vi "ChipScope Control.vi"() -> ()   [LabVIEW 2017]
uses:
  <instrlib>/TLDC4100/TLDC4100.llb/z_StateMachineVorlage.ctl
  C:/Program Files/National Instruments/LabVIEW 2017/instr.lib/IDS/ueye.NET/uEyeDotNet.dll
panel:
  in  "Acquisition tab":enum32{"Acquisition", "Bookmarks"}(tab)
  in  "Exposure 3":dbl=100.0
  in  "Exposure 2":dbl=100.0
  in  "Gain 3":i32=100 min=100 max=2000
  in  "Gain 2":i32=100 min=100 max=2000
  in  "Gain 1":i32=100 caption="Gain" min=100 max=2000
  in  "Exposure 1":dbl=100.0 caption="Exp."
  in  "Acq. order":string(combo)="3"
  in  "ACQUIRE":bool
  in  "Autosave?":bool
  in  "Use bookmarks?":bool
  in  "t-delay (ms)":dbl min=0.0 max=75.0
  in  "# t-frames":i32=1 min=0 max=75
  in  "z-step (um)":dbl=1.0 min=0.0 max=75.0
  in  "# z-steps":i32=1 min=0 max=75
  in  "3:":string(combo)="99"
  in  "2:":string(combo)="99"
  in  "1:":string(combo)="0"
  in  "Illumination tab":enum32{"Laser power", "LED power"}(tab)
  in  "Red power":dbl=1.0 min=0.0 max=120.0
  in  "Green power":dbl=1.0 min=0.0 max=150.0
  in  "Blue power":dbl=1.0 min=0.0 max=150.0
  in  "445 power":dbl=1.0 min=0.0 max=75.0
  in  "Illumination":bool
  out "Live":bool
  in  "Gain":i32=100 min=100 max=2000
  in  "Exposure (ms)":dbl=100.0
  in  "Live channel":enum8{"Red", "Green", "Blue"}(ring)
  in  "LIVE":bool
  out "Image":T1(plugin-control)
  out "Status":string
  out "Connected":bool
  out "error out":errorcluster
  in  "Quit":bool
  in  "error in":errorcluster
  out "State":T2 caption="States"
  # "Laser"
  # "LEDs"
  # "Laser power"
  # "Debugging area"
  # "Channel order"
  # "Acquisition order"
  # "LEDs seem to have a\nproblem with the \ndriver hardware at the\nmoment!! :("
  # "mW"
  # "mW"
  # "mW"
  # "mW"
  # "LEDs seem to have a\nproblem with the \ndriver hardware at the\nmoment!! :("
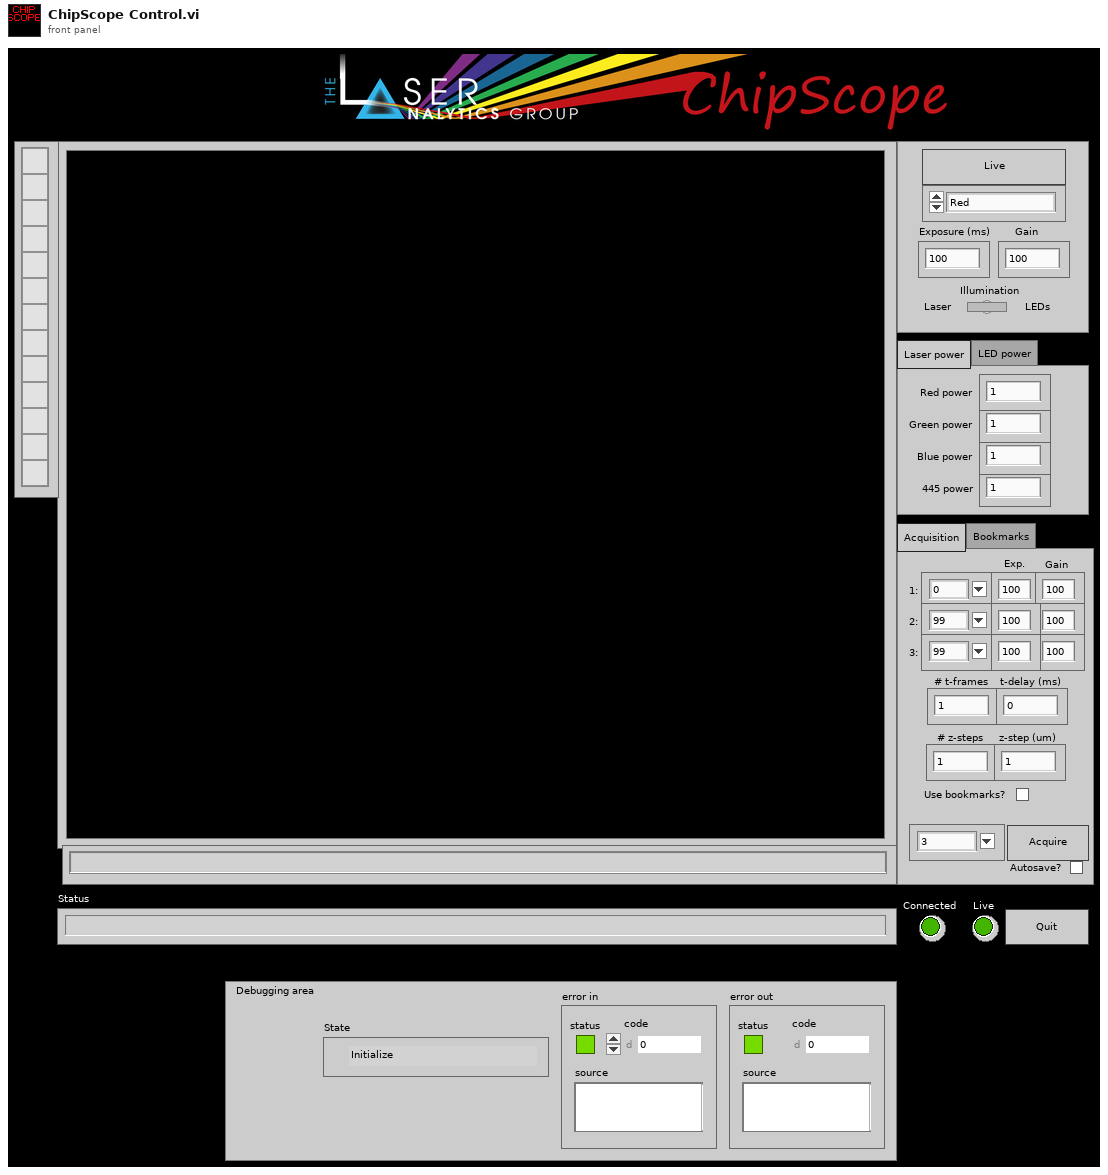
[diagram p1: front panel]
types:
  T1 = typedef "IMAQ Image.ctl" = refnum<image>
  T2 = typedef "z_StateMachineVorlage.ctl" = enum16{"Initialize", "1", "2", "3", "4", "5", "6", "7", "8", "9", "10", "11", "12", "13", "14", "15", "20", "25", "30", "35", "40", "45", "50", "55", "59", "60", "65", "70", "75", "76", "77", "78", "79", "80", "85", "90", "91", "92", "93", "94", "95", "96", "97", "98", "99", "100", "105", "110", "120", "130", "140", "150", "160", "170", "180", "190", "200", "201", "205", "210", "215", "220", "230", "240", "245", "250", "255", "260", "270", "280", "290", "300", "310", "313", "315", "318", "320", "330", "340", "350", "360", "370", "380", "390", "400", "410", "420", "430", "440", "450", "460", "470", "480", "490", "500", "501", "502", "510", "520", "523", "525", "528", "530", "540", "550", "560", "570", "580", "590", "600", "605", "610", "620", "630", "640", "650", "660", "670", "680", "690", "700", "710", "720", "730", "740", "750", "760", "770", "780", "790", "800", "810", "820", "830", "840", "850", "860", "870", "880", "890", "900", "910", "920", "930", "940", "950", "960", "970", "980", "990", "1000", "1010", "1020", "1030", "1040", "1050", "1060", "1070", "1080", "1090", "1100", "1110", "1120", "1130", "1140", "1150", "1160", "1170", "1180", "1190", "1200", "1210", "1220", "1230", "1240", "1250", "1260", "1270", "1280", "1290", "1300", "1310", "1320", "1330", "1340", "1350", "1360", "1370", "1380", "1390", "1400", "1410", "1420", "1430", "1440", "1450", "1460", "1470", "1480", "1490", "1500", "Fehler I", "Fehler II", "Fehler III", "Fehler IV", "Fehler V", "Fehler VI", "Fehler VII", "Fehler VIII", "Fehler IX", "Fehler X", "Stop"}
  T3 = cluster{"Save path":path, "t frame":i32, "bookmark #":i32, "Z-step":i32, "Channel":i32, "total t frames":i32, "Total bookmarks":i32, "Total z steps":i32, "Total channels":i32}
  T4 = cluster{"LED handle":refnum<visa-resource-name>, "Laser cluster":cluster{"445 laser":refnum<visa-resource-name>, "488 laser":refnum<visa-resource-name>, "561 laser":refnum<visa-resource-name>, "640 laser":refnum<visa-resource-name>}, "Piezo handle":i32, "Camera cluster":cluster{"Red camera":refnum<k24>, "Green camera":refnum<k24>, "Blue camera":refnum<k24>}}
  T5 = cluster{"445 laser":refnum<visa-resource-name>, "488 laser":refnum<visa-resource-name>, "561 laser":refnum<visa-resource-name>, "640 laser":refnum<visa-resource-name>}
  T6 = cluster{"Red camera":refnum<k24>, "Green camera":refnum<k24>, "Blue camera":refnum<k24>}
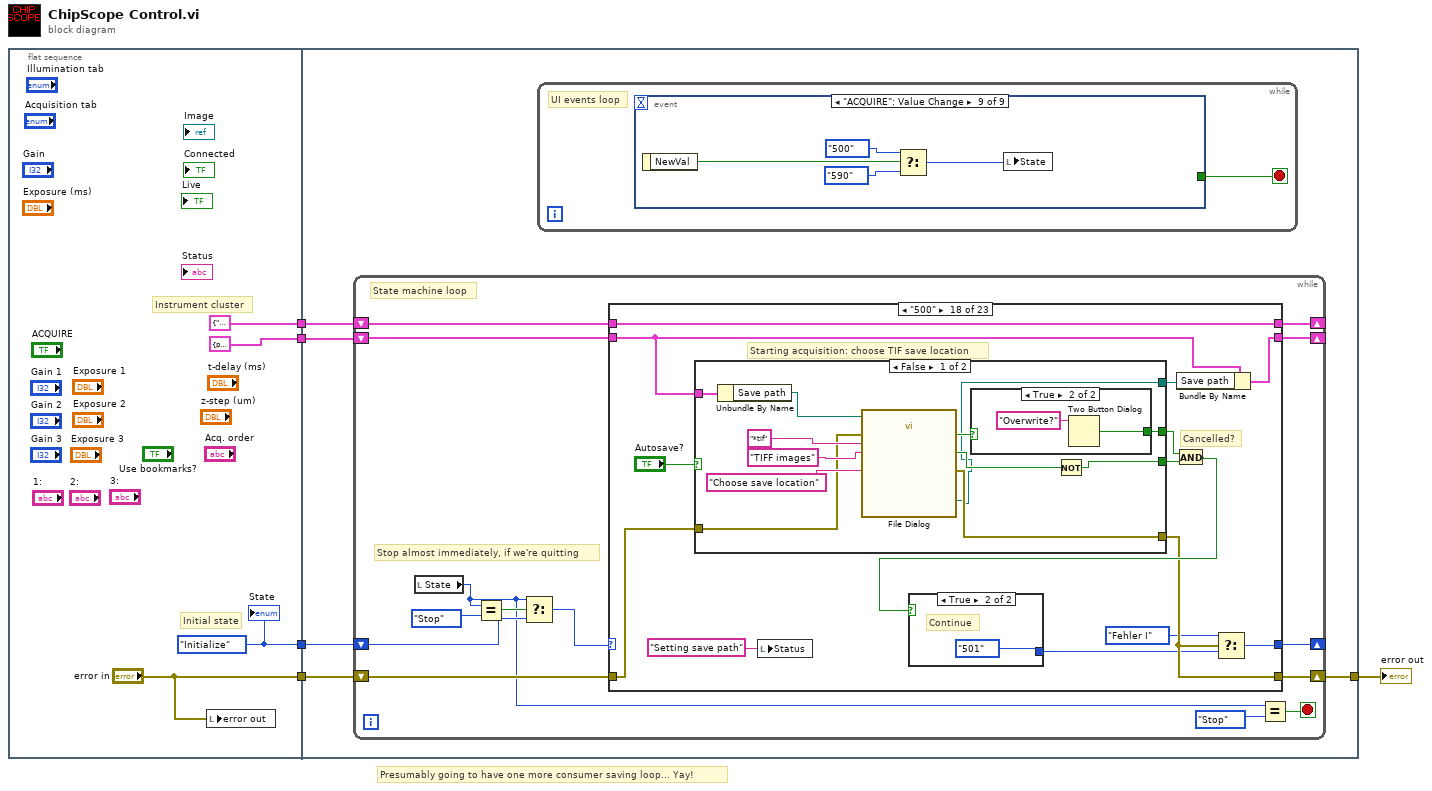
[diagram p0: block diagram]
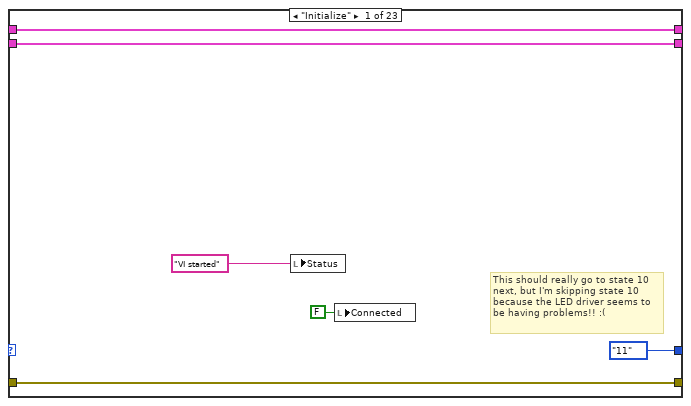
[diagram p2: hidden frame]
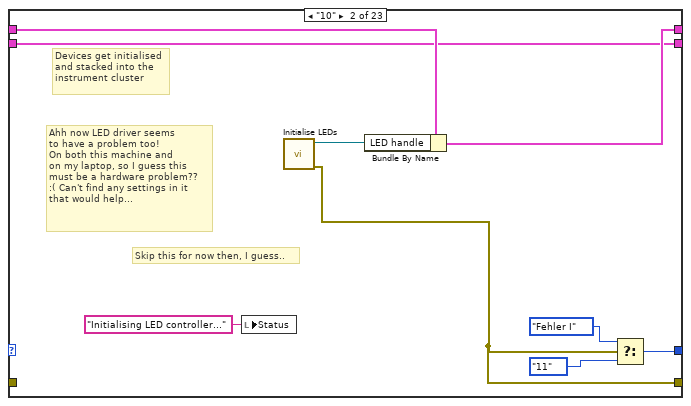
[diagram p3: hidden frame]
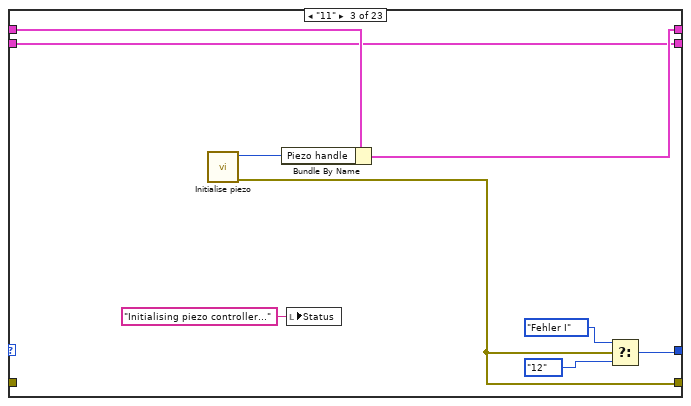
[diagram p4: hidden frame]
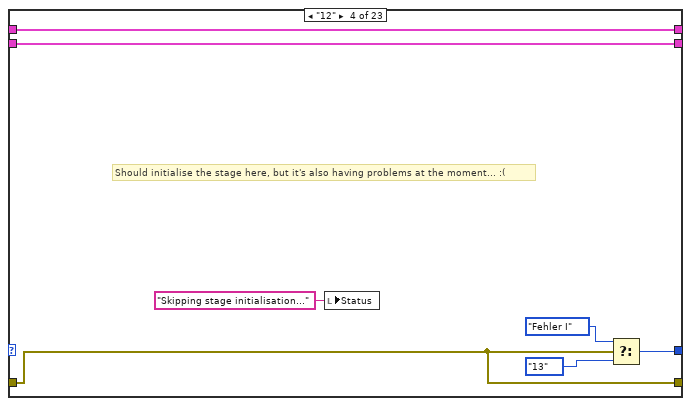
[diagram p5: hidden frame]
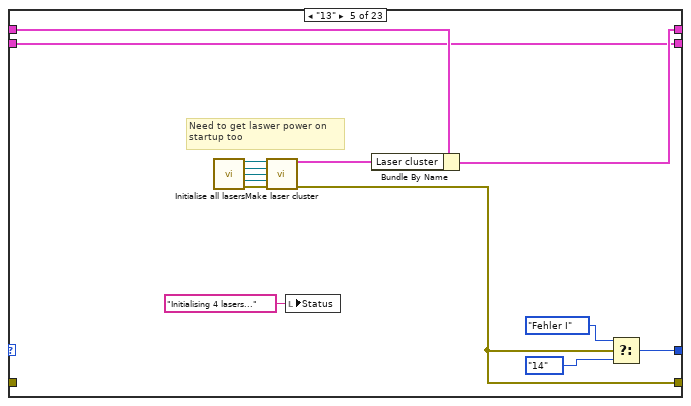
[diagram p6: hidden frame]
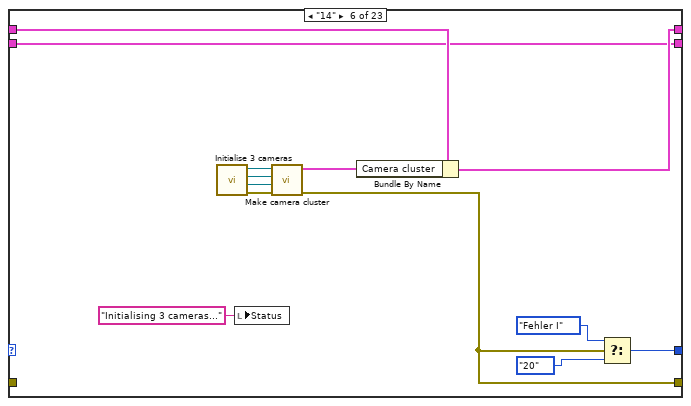
[diagram p7: hidden frame]
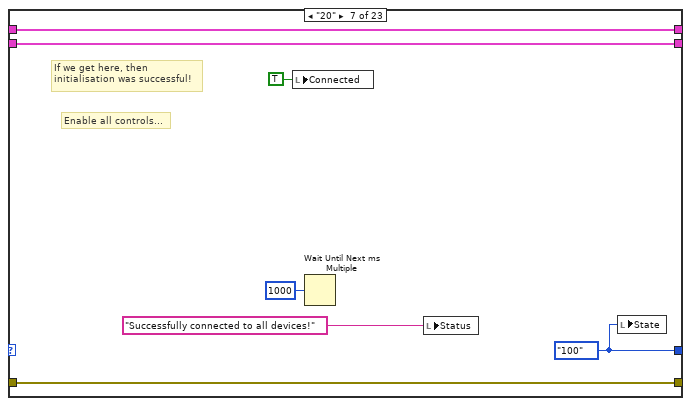
[diagram p8: hidden frame]
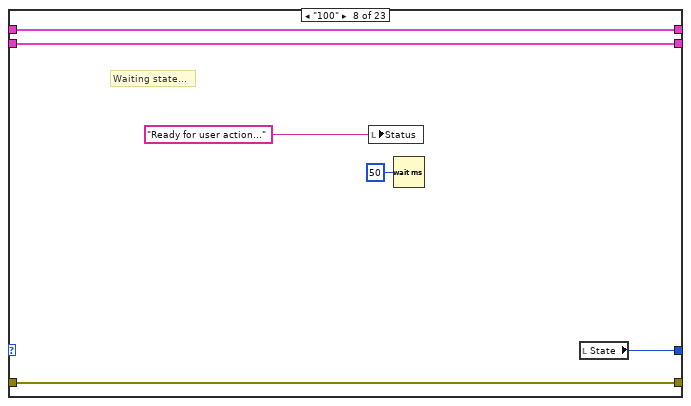
[diagram p9: hidden frame]
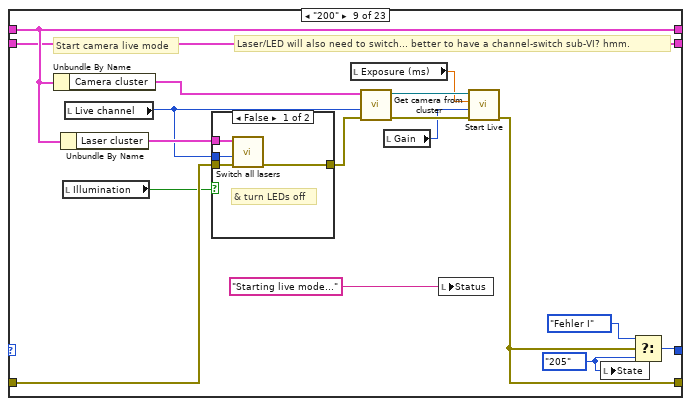
[diagram p10: hidden frame]
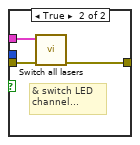
[diagram p11: hidden frame]
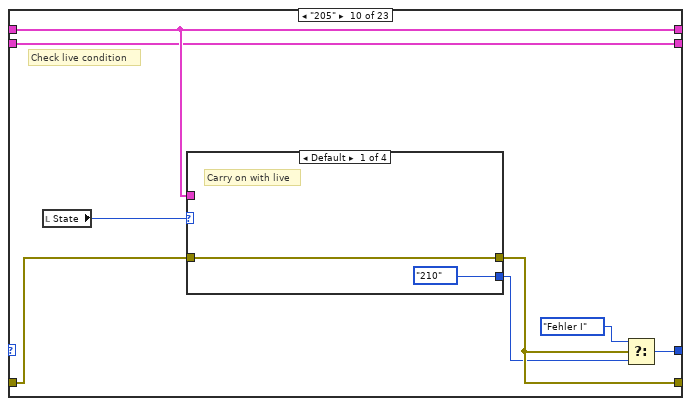
[diagram p12: hidden frame]
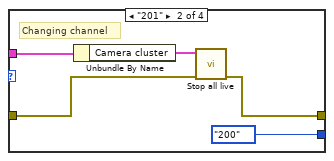
[diagram p13: hidden frame]
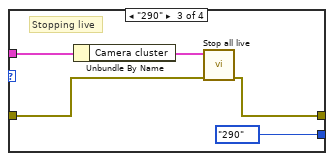
[diagram p14: hidden frame]
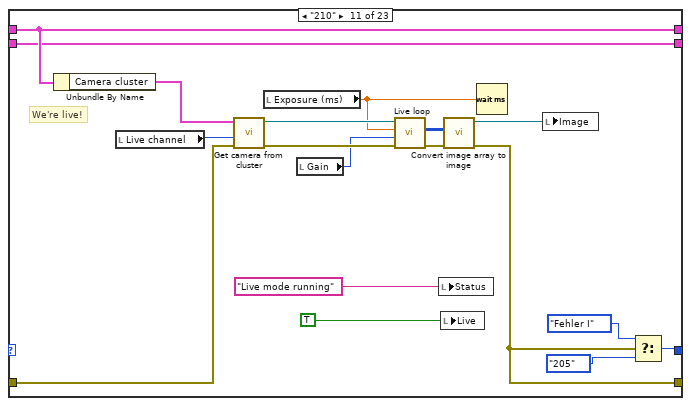
[diagram p16: hidden frame]
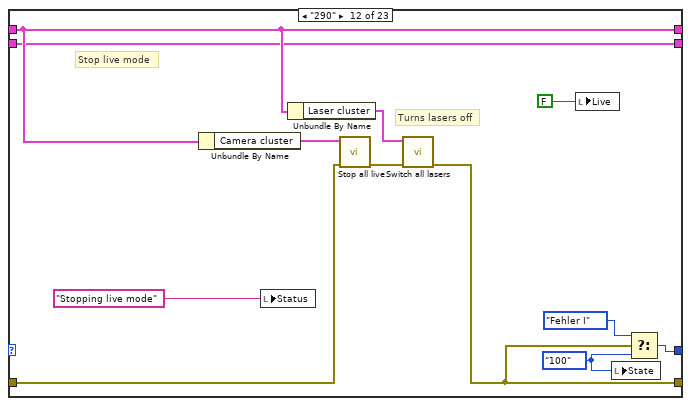
[diagram p17: hidden frame]
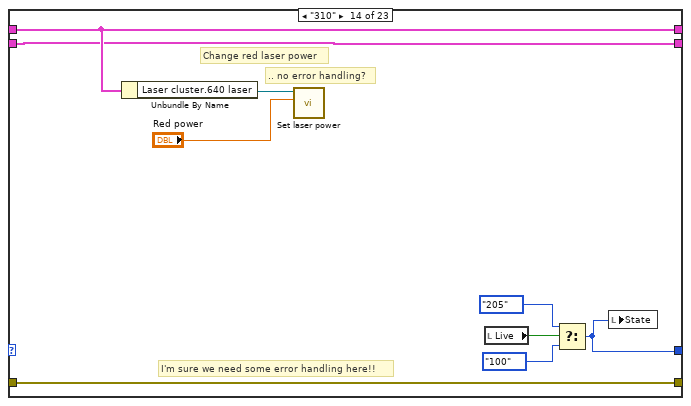
[diagram p19: hidden frame]
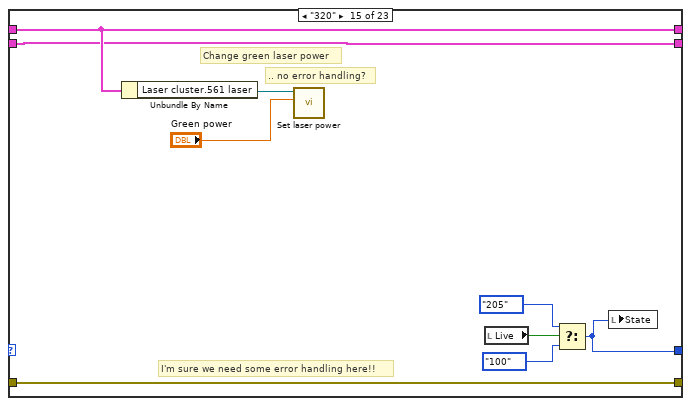
[diagram p20: hidden frame]
diagram:
  # "Presumably going to have one more consumer saving loop... Yay!"
  n1 = flat-sequence {
    tunnel: [T4 {"LED handle"="", "Laser cluster"={"445 laser"="", "488 laser"="", "561 laser"="", "640 laser"=""}, "Piezo handle"=0, "Camera cluster"={"Red camera"=refnum, "Green camera"=refnum, "Blue camera"=refnum}} ("Instrument cluster")] -> w5
    tunnel: ["error in"] -> w3
    tunnel: [w7] -> w2
    tunnel: [T3 {"Save path"=path "D:/DATA_2018", "t frame"=0, "bookmark #"=0, "Z-step"=0, "Channel"=0, "total t frames"=0, "Total bookmarks"=0, "Total z steps"=0, "Total channels"=0} ("Instrument cluster")] -> w1
    tunnel: w5 -> [w14]
    tunnel: [w13] -> w4
    tunnel: w3 -> [w12]
    tunnel: w2 -> [w11]
    tunnel: w1 -> [w10]
    frame #0 {
      w7 = z_StateMachineVorlage."Initialize" ("States")
      # "Initial state"
      # "Instrument cluster"
      n2 = local write "error out"("error in") -> ()
      "State" <- w7
    }
    frame #1 {
      n3 = while {
        shift-right: [w28] -> _
        shift-left: w11 -> [w18]
        shift-right: [w25] -> _
        shift-left: w14 -> [w22]
        shift-right: [w24] -> w13
        shift-left: w12 -> [w23]
        shift-right: [w16] -> _
        shift-left: w10 -> [w15]
        stop <- w27 stop-if-true
        # "State machine loop"
        # "Stop almost immediately, if we're quitting"
        n4 = local read "State"() -> (w17:T2)
        n5 = Equal?(x=w17, y=z_StateMachineVorlage."Stop" ("States")) -> (x = y?=w20:bool)
        n6 = Select(t=w17, s=w20, f=w18) -> (s? t:f=w19:T2)
        n7 = case shown="\"500\"" w19 {
          selector: w19 -> [_ _ _ _ _ _ _ _ _ _ _ _ w179 _ _ _ _ _ _ _ w290 _ _]
          tunnel: [z_StateMachineVorlage."11" ("States") w41 w47 w56 w62 w75 w88 w95 w114 w128 w160 w172 w179 w181 w191 w200 w209 w221 z_StateMachineVorlage."502" ("States") _ w290 z_StateMachineVorlage."Stop" ("States") z_StateMachineVorlage."900" ("States")] -> w28
          tunnel: [w31 w37 w51 w54 w64 w79 w90 w99 w106 w131 w163 w166 w177 w188 w197 w206 w215 w229 w261 w284 w289 w296 w302] -> w25
          tunnel: w22 -> [w31 w36 w50 w54 w65 w80 w90 w99 w106 w131 w163 w166 w177 w188 w197 w206 w215 w229 w261 w284 w289 w296 w302]
          tunnel: [w32 w39 w46 w55 w63 w76 w91 w97 w115 w127 w149 w168 w178 w182 w192 w201 w210 w223 w250 w276 w291 w293 w311] -> w24
          tunnel: w23 -> [w32 _ _ w55 _ _ w91 w97 w103 w130 w157 w175 w178 w182 w192 w201 w210 w227 w250 w276 w291 w294 w300]
          tunnel: w15 -> [w29 w35 w44 w53 w60 w74 w87 w94 w100 w124 w146 w164 w176 w180 w189 w198 w207 w218 w265 w285 w288 w292 w297]
          tunnel: [w29 w35 w44 w53 w60 w74 w87 w94 w100 w124 w146 w164 w176 w180 w189 w198 w207 w217 w253 w277 w288 w292 w297] -> w16
          frame "Initialize" {
            # "This should really go to state 10\nnext, but I'm skipping state 10\nbecause the LED driver seems to\nbe having problems!! :("
            n8 = local write "Status"("VI started" ("Status")) -> ()
            n9 = local write "Connected"(FALSE ("Connected")) -> ()
          }
          frame "10" {
            # "Skip this for now then, I guess.."
            # "Ahh now LED driver seems\nto have a problem too!\nOn both this machine and \non my laptop, so I guess this\nmust be a hardware problem??\n:( Can't find any settings in it \nthat would help..."
            # "Devices get initialised\nand stacked into the\ninstrument cluster"
            n10 = local write "Status"("Initialising LED controller..." ("Status")) -> ()
            n11 = call "Initialise LEDs.vi"() -> ("error out"=w39:errorcluster, "LED handle"=w38:refnum<visa-resource-name>)  [unwired: 10 in]
            n12 = Bundle By Name(cluster=w36, "LED handle"=w38) -> (w37:T4)
            n13 = Select(t=z_StateMachineVorlage."Fehler I", s=w39, f=z_StateMachineVorlage."11" ("States")) -> (s? t:f=w41:T2)
          }
          frame "11" {
            n14 = call "Initialise piezo.vi"() -> ("Piezo error out"=w46:errorcluster, "Piezo handle"=w52:i32)  [unwired: 10 in]
            n15 = Bundle By Name(cluster=w50, "Piezo handle"=w52) -> (w51:T4)
            n16 = local write "Status"("Initialising piezo controller..." ("Status")) -> ()
            n17 = Select(t=z_StateMachineVorlage."Fehler I", s=w46, f=z_StateMachineVorlage."12" ("States")) -> (s? t:f=w47:T2)
          }
          frame "12" {
            # "Should initialise the stage here, but it's also having problems at the moment... :("
            n18 = local write "Status"("Skipping stage initialisation..." ("Status")) -> ()
            n19 = Select(t=z_StateMachineVorlage."Fehler I", s=w55, f=z_StateMachineVorlage."13" ("States")) -> (s? t:f=w56:T2)
          }
          frame "13" {
            # "Need to get laswer power on \nstartup too"
            n20 = call "Initialise all lasers.vi"() -> ("455 laser"=w71:refnum<visa-resource-name>, "488 laser"=w70:refnum<visa-resource-name>, "561 laser"=w69:refnum<visa-resource-name>, "647 laser"=w68:refnum<visa-resource-name>, "error out"=w67:errorcluster)  [unwired: 11 in]
            n21 = call "Make laser cluster.vi"("445 laser"=w71, "488 laser"=w70, "561 laser"=w69, "640 laser"=w68, "Error In"=w67) -> ("Laser cluster"=w66:T5, "Error Out"=w63:errorcluster)  [unwired: 9 in]
            n22 = local write "Status"("Initialising 4 lasers..." ("Status")) -> ()
            n23 = Bundle By Name(cluster=w65, "Laser cluster"=w66) -> (w64:T4)
            n24 = Select(t=z_StateMachineVorlage."Fehler I", s=w63, f=z_StateMachineVorlage."14" ("States")) -> (s? t:f=w62:T2)
          }
          frame "14" {
            n25 = call "Initialise 3 cameras.vi"() -> ("Error Out"=w83:errorcluster, "Blue camera ref"=w84:refnum<k24>, "Green camera ref"=w85:refnum<k24>, "Red camera ref"=w86:refnum<k24>)  [unwired: 8 in]
            n26 = local write "Status"("Initialising 3 cameras..." ("Status")) -> ()
            n27 = call "Make camera cluster.vi"("Error In"=w83, "Blue ref"=w84, "Green ref"=w85, "Red ref"=w86) -> ("Error Out"=w76:errorcluster, "Camera cluster"=w81:T6)  [unwired: 6 in]
            n28 = Bundle By Name(cluster=w80, "Camera cluster"=w81) -> (w79:T4)
            n29 = Select(t=z_StateMachineVorlage."Fehler I", s=w76, f=z_StateMachineVorlage."20" ("States")) -> (s? t:f=w75:T2)
          }
          frame "20" {
            w88 = z_StateMachineVorlage."100" ("States")
            # "Enable all controls..."
            # "If we get here, then \ninitialisation was successful!"
            n30 = local write "Connected"(TRUE ("Connected")) -> ()
            n31 = Wait Until Next ms Multiple(millisecond multiple=u32 1000) -> ()  [unwired: 1 out]
            n32 = local write "Status"("Successfully connected to all devices!" ("Status")) -> ()
            n33 = local write "State"(w88) -> ()
          }
          frame "100" {
            # "Waiting state..."
            n34 = local write "Status"("Ready for user action..." ("Status")) -> ()
            n35 = Wait (ms)(milliseconds to wait=u32 50) -> ()  [unwired: 1 out]
            n36 = local read "State"() -> (w95:T2)
          }
          frame "200" {
            w107 = z_StateMachineVorlage."205" ("States")
            # "Laser/LED will also need to switch... better to have a channel-switch sub-VI? hmm."
            # "Start camera live mode"
            n37 = Unbundle By Name(w106) -> ("Camera cluster"=w113:T6)
            n38 = Unbundle By Name(w106) -> ("Laser cluster"=w105:T5)
            n39 = local read "Illumination"() -> (w101:bool)
            n40 = local read "Live channel"() -> (w104:enum8{"Red", "Green", "Blue"})
            n41 = case shown="False" w101 {
              tunnel: w105 -> [w120 w123]
              tunnel: w104 -> [w119 _]
              tunnel: w103 -> [w118 w122]
              tunnel: [w117 w121] -> w102
              frame False {
                # "& turn LEDs off"
                n42 = call "Switch all lasers.vi"("error in"=w118, "Live channel"=w119, "Laser cluster"=w120) -> ("error out"=w117:errorcluster)  [unwired: 8 in]
              }
              frame True {
                # "& switch LED \nchannel..."
                n43 = call "Switch all lasers.vi"("error in"=w122, "Laser cluster"=w123) -> ("error out"=w121:errorcluster)  [unwired: 9 in]
              }
            }
            n44 = local read "Exposure (ms)"() -> (w109:dbl)
            n45 = call "Get camera from cluster.vi"("Error In"=w102, "Camera"=w104, "Camera cluster"=w113) -> ("Error Out"=w111:errorcluster, "Camera reference out"=w112:refnum<k24>)  [unwired: 7 in]
            n46 = local read "Gain"() -> (w110:i32)
            n47 = local write "Status"("Starting live mode..." ("Status")) -> ()
            n48 = call "Start Live.vi"("Error In"=w111, "Gain in"=w110, "Exposure time (ms)"=w109, "Camera reference in"=w112) -> ("Error Out"=w115:errorcluster)  [unwired: 5 in, 1 out]
            n49 = local write "State"(w107) -> ()
            n50 = Select(t=z_StateMachineVorlage."Fehler I", s=w115, f=w107) -> (s? t:f=w114:T2)
          }
          frame "205" {
            # "Check live condition"
            n51 = local read "State"() -> (w126:T2)
            n52 = case shown="Default" w126 {
              selector: w126 -> [_ _ _ w145]
              tunnel: w131 -> [_ w138 w143 _]
              tunnel: w130 -> [w133 w136 w141 w144]
              tunnel: [w133 w135 w140 w144] -> w127
              tunnel: [z_StateMachineVorlage."210" ("States") z_StateMachineVorlage."200" ("State") z_StateMachineVorlage."290" ("State") w145] -> w125
              frame Default {
                # "Carry on with live"
              }
              frame "201" {
                # "Changing channel"
                n53 = Unbundle By Name(w138) -> ("Camera cluster"=w137:T6)
                n54 = call "Stop all live.vi"("Error In"=w136, "Camera cluster"=w137) -> ("Error Out"=w135:errorcluster)  [unwired: 8 in]
              }
              frame "290" {
                # "Stopping live"
                n55 = Unbundle By Name(w143) -> ("Camera cluster"=w142:T6)
                n56 = call "Stop all live.vi"("Error In"=w141, "Camera cluster"=w142) -> ("Error Out"=w140:errorcluster)  [unwired: 8 in]
              }
              frame "310", "320".."340" {
                # "Changing laser powers"
              }
            }
            n57 = Select(t=z_StateMachineVorlage."Fehler I", s=w127, f=w125) -> (s? t:f=w128:T2)
          }
          frame "210" {
            # "We're live!"
            n58 = Unbundle By Name(w163) -> ("Camera cluster"=w159:T6)
            n59 = local read "Live channel"() -> (w158:enum8{"Red", "Green", "Blue"})
            n60 = call "Get camera from cluster.vi"("Error In"=w157, "Camera"=w158, "Camera cluster"=w159) -> ("Error Out"=w155:errorcluster, "Camera reference out"=w153:refnum<k24>)  [unwired: 7 in]
            n61 = local read "Exposure (ms)"() -> (w147:dbl)
            n62 = local read "Gain"() -> (w154:i32)
            n63 = call "Live loop.vi"("Error In"=w155, "Gain"=w154, "Exposure time (ms)"=w147, "Camera reference in"=w153) -> ("Error Out"=w152:errorcluster, "Image Array"=w151:u16[][])  [unwired: 4 in, 1 out]
            n64 = local write "Status"("Live mode running" ("Status")) -> ()
            n65 = local write "Live"(TRUE ("Live")) -> ()
            n66 = call "Convert image array to image.vi"("Error In"=w152, "Array"=w151) -> ("error out"=w149:errorcluster, "Image Out"=w150:T1)  [unwired: 7 in]
            n67 = Wait (ms)(milliseconds to wait=w147) -> ()  [unwired: 1 out]
            n68 = local write "Image"(w150) -> ()
            n69 = Select(t=z_StateMachineVorlage."Fehler I", s=w149, f=z_StateMachineVorlage."205" ("States")) -> (s? t:f=w160:T2)
          }
          frame "290" {
            w165 = z_StateMachineVorlage."100" ("States")
            # "Turns lasers off"
            # "Stop live mode"
            n70 = Unbundle By Name(w166) -> ("Camera cluster"=w174:T6)
            n71 = local write "Status"("Stopping live mode" ("Status")) -> ()
            n72 = Unbundle By Name(w166) -> ("Laser cluster"=w167:T5)
            n73 = call "Stop all live.vi"("Error In"=w175, "Camera cluster"=w174) -> ("Error Out"=w169:errorcluster)  [unwired: 8 in]
            n74 = call "Switch all lasers.vi"("error in"=w169, "Laser cluster"=w167) -> ("error out"=w168:errorcluster)  [unwired: 9 in]
            n75 = local write "Live"(FALSE ("Live")) -> ()
            n76 = local write "State"(w165) -> ()
            n77 = Select(t=z_StateMachineVorlage."Fehler I", s=w168, f=w165) -> (s? t:f=w172:T2)
          }
          frame "300" {
          }
          frame "310" {
            # "I'm sure we need some error handling here!!"
            # ".. no error handling?"
            # "Change red laser power"
            n78 = Unbundle By Name(w188) -> ("Laser cluster.640 laser"=w187:refnum<visa-resource-name>)
            n79 = call "Set laser power.vi"("Laser Power"="Red power", "VISA resource name"=w187) -> ()  [unwired: 9 in, 1 out]
            n80 = local read "Live"() -> (w185:bool)
            n81 = Select(t=z_StateMachineVorlage."205" ("States"), s=w185, f=z_StateMachineVorlage."100" ("States")) -> (s? t:f=w181:T2)
            n82 = local write "State"(w181) -> ()
          }
          frame "320" {
            # "I'm sure we need some error handling here!!"
            # ".. no error handling?"
            # "Change green laser power"
            n83 = Unbundle By Name(w197) -> ("Laser cluster.561 laser"=w196:refnum<visa-resource-name>)
            n84 = call "Set laser power.vi"("Laser Power"="Green power", "VISA resource name"=w196) -> ()  [unwired: 9 in, 1 out]
            n85 = local read "Live"() -> (w195:bool)
            n86 = Select(t=z_StateMachineVorlage."205" ("States"), s=w195, f=z_StateMachineVorlage."100" ("States")) -> (s? t:f=w191:T2)
            n87 = local write "State"(w191) -> ()
          }
          frame "330" {
            # "I'm sure we need some error handling here!!"
            # ".. no error handling?"
            # "Change blue laser power"
            n88 = Unbundle By Name(w206) -> ("Laser cluster.488 laser"=w205:refnum<visa-resource-name>)
            n89 = call "Set laser power.vi"("Laser Power"="Blue power", "VISA resource name"=w205) -> ()  [unwired: 9 in, 1 out]
            n90 = local read "Live"() -> (w204:bool)
            n91 = Select(t=z_StateMachineVorlage."205" ("States"), s=w204, f=z_StateMachineVorlage."100" ("States")) -> (s? t:f=w200:T2)
            n92 = local write "State"(w200) -> ()
          }
          frame "340" {
            # "I'm sure we need some error handling here!!"
            # ".. no error handling?"
            # "Change 445 laser power"
            n93 = Unbundle By Name(w215) -> ("Laser cluster.445 laser"=w214:refnum<visa-resource-name>)
            n94 = call "Set laser power.vi"("Laser Power"="445 power", "VISA resource name"=w214) -> ()  [unwired: 9 in, 1 out]
            n95 = local read "Live"() -> (w213:bool)
            n96 = Select(t=z_StateMachineVorlage."205" ("States"), s=w213, f=z_StateMachineVorlage."100" ("States")) -> (s? t:f=w209:T2)
            n97 = local write "State"(w209) -> ()
          }
          frame "500" {
            # "Cancelled?"
            # "Starting acquisition: choose TIF save location"
            n98 = case shown="False" "Autosave?" {
              tunnel: w227 -> [w240 w249]
              tunnel: [w239 w249] -> w223
              tunnel: [w236 w248] -> w226
              tunnel: [w237 w248] -> w225
              tunnel: w218 -> [w234 _]
              tunnel: [w232 path "D:/DATA_2018/test.tif" ("selected path")] -> w219
              frame False {
                n99 = Unbundle By Name(w234) -> ("Save path"=w233:path)
                n100 = call "File Dialog"("start path"=w233, "prompt"="Choose save location", "error in"=w240, "pattern (all files)"="*tif", "pattern label"="TIFF images") -> ("selected path"=w232:path, "exists"=w238:bool, "cancelled"=w235:bool, "error out"=w239:errorcluster)  [unwired: 7 in]
                n101 = case shown="True" w238 {
                  tunnel: [TRUE ("T button?") w245] -> w237
                  frame False {
                  }
                  frame True {
                    n102 = Two Button Dialog(message="Overwrite?") -> (T button?=w245:bool)  [unwired: 2 in]
                  }
                }
                n103 = Not(x=w235) -> (.not. x?=w236:bool)
              }
              frame True {
                w248 = TRUE ("T button?")
                # "Err.. need to implement this..."
              }
            }
            n104 = local write "Status"("Setting save path" ("Status")) -> ()
            n105 = And(x=w225, y=w226) -> (x .and. y?=w224:bool)
            n106 = case shown="True" w224 {
              tunnel: [z_StateMachineVorlage."100" ("States") z_StateMachineVorlage."501" ("States")] -> w222
              frame False {
                # "Cancelled"
              }
              frame True {
                # "Continue"
              }
            }
            n107 = Bundle By Name(cluster=w218, "Save path"=w219) -> (w217:T3)
            n108 = Select(t=z_StateMachineVorlage."Fehler I", s=w223, f=w222) -> (s? t:f=w221:T2)
          }
          frame "501" {
            # "Need to make bookmarking capability"
            n109 = local read "1:"() -> (w260:string)
            n110 = Bundle By Name(cluster=w265, "total t frames"="# t-frames") -> (w262:T3)
            n111 = case shown="Default" w260 {
              tunnel: 0 -> [w274 w275]
              tunnel: [w273 w275] -> w256
              frame Default {
                n112 = Increment(x=w274) -> (x+1=w273:i32)
              }
              frame "None" {
              }
            }
            n113 = Bundle By Name(cluster=w262, "Total z steps"="# z-steps") -> (w252:T3)
            n114 = local read "2:"() -> (w257:string)
            n115 = local write "Status"("Setting acquisition parameters" ("Status")) -> ()
            n116 = case shown="Default" w257 {
              tunnel: w256 -> [w271 w272]
              tunnel: [w270 w272] -> w255
              frame Default {
                n117 = Increment(x=w271) -> (x+1=w270:i32)
              }
              frame "None" {
              }
            }
            n118 = local read "3:"() -> (w258:string)
            n119 = case shown="\"None\"" w258 {
              tunnel: w255 -> [w268 w269]
              tunnel: [w267 w269] -> w254
              frame Default {
                n120 = Increment(x=w268) -> (x+1=w267:i32)
              }
              frame "None" {
              }
            }
            n121 = Bundle By Name(cluster=w252, "Total channels"=w254) -> (w253:T3)
          }
          frame "502" {
            n122 = Bundle By Name(cluster=w285, "t frame"=0) -> (w280:T3)
            n123 = Bundle By Name(cluster=w280, "bookmark #"=0 ("t frame")) -> (w279:T3)
            n124 = Bundle By Name(cluster=w279, "Z-step"=0 ("t frame")) -> (w278:T3)
            n125 = Bundle By Name(cluster=w278, "Channel"=0 ("t frame")) -> (w277:T3)
            n126 = local write "Status"("Resetting acquisition status" ("Status")) -> ()
          }
          frame "900" {
            # "A state where nothing happens."
          }
          frame "Fehler I" {
            # "Handle errors"
            n127 = call <vilib>:"Simple Error Handler.vi"("error in (no error)"=w294) -> ("error out"=w293:errorcluster)  [unwired: 4 in, 4 out]
          }
          frame "Stop", Default {
            # "Don't error check on\nStop, or we'll get into\na loop..."
            # "Will need to close\nLEDs when we have \nthem working again"
            # "Shut everything down safely"
            n128 = Unbundle By Name(w302) -> ()  [unwired: 1 out]
            n129 = Unbundle By Name(w302) -> ("Laser cluster"=w309:T5)
            n130 = Select(t="Please quit the VI. A fatal error occured and buttons will now be unresponsive. ", s=w300, f="Stopping VI" ("Status")) -> (s? t:f=w308:string)
            n131 = local write "Connected"(FALSE ("Connected")) -> ()
            n132 = call "Close all lasers.vi"("error in"=w300, "Laser cluster"=w309) -> ("error out"=w312:errorcluster)  [unwired: 9 in]
            n133 = Unbundle By Name(w302) -> ("Piezo handle"=w310:i32)
            n134 = local write "Status"(w308) -> ()
            n135 = Unbundle By Name(w302) -> ("Camera cluster"=w301:T6)
            n136 = call "Close piezo.vi"("Piezo error in"=w312, "Piezo handle"=w310) -> ("error out"=w304:errorcluster)  [unwired: 9 in]
            n137 = call "Stop all live.vi"("Error In"=w304, "Camera cluster"=w301) -> ("Error Out"=w303:errorcluster)  [unwired: 8 in]
            n138 = call "Close stage.vi"("error in"=w303) -> ("error out"=w311:errorcluster)  [unwired: 10 in]
            n139 = local write "LIVE"(FALSE ("Live")) -> ()
            n140 = local write "Live"(FALSE ("Live")) -> ()
          }
        }
        n141 = Equal?(x=w17, y=z_StateMachineVorlage."Stop" ("States")) -> (x = y?=w27:bool)
      }
      n142 = while {
        stop <- w314 stop-if-true
        # "UI events loop"
        n143 = event shown="[8] \"ACQUIRE\": Value Change" {
          selector: _ -> [_ _ _ _ _ _ _ _ _]
          dyn-events: _ -> [_ _ _ _ _ _ _ _ _]
          timeout: _ -> [_ _ _ _ _ _ _ _ _]
          tunnel: [_ w316 _ _ _ _ _ _ _] -> w314
          event Timeout {
            n144 = event-data() -> ()  [unwired: 1 in, 1 out]
          }
          event "Quit": Value Change {
            n145 = event-data() -> ("NewVal"=w316:bool)  [unwired: 1 in]
            n146 = local write "State"(z_StateMachineVorlage."Stop" ("States")) -> ()
          }
          event "LIVE": Value Change {
            n147 = event-data() -> ("NewVal"=w320:bool)  [unwired: 1 in]
            n148 = Select(t=z_StateMachineVorlage."200" ("States"), s=w320, f=z_StateMachineVorlage."290" ("States")) -> (s? t:f=w319:T2)
            n149 = local write "State"(w319) -> ()
          }
          event "Live channel", "Illumination": Value Change {
            n150 = event-data() -> ()  [unwired: 1 in, 1 out]
            n151 = local read "Live"() -> (w321:bool)
            n152 = case shown="True" w321 {
              frame False {
              }
              frame True {
                n153 = local write "State"(z_StateMachineVorlage."201" ("State")) -> ()
              }
            }
          }
          event "Red power": Value Change {
            n154 = event-data() -> ()  [unwired: 1 in, 1 out]
            n155 = local write "State"(z_StateMachineVorlage."310" ("State")) -> ()
          }
          event "Green power": Value Change {
            n156 = event-data() -> ()  [unwired: 1 in, 1 out]
            n157 = local write "State"(z_StateMachineVorlage."320" ("State")) -> ()
          }
          event "Blue power": Value Change {
            n158 = event-data() -> ()  [unwired: 1 in, 1 out]
            n159 = local write "State"(z_StateMachineVorlage."330" ("State")) -> ()
          }
          event "445 power": Value Change {
            n160 = event-data() -> ()  [unwired: 1 in, 1 out]
            n161 = local write "State"(z_StateMachineVorlage."340" ("State")) -> ()
          }
          event "ACQUIRE": Value Change {
            n162 = event-data() -> ("NewVal"=w327:bool)  [unwired: 1 in]
            n163 = Select(t=z_StateMachineVorlage."500" ("States"), s=w327, f=z_StateMachineVorlage."590" ("States")) -> (s? t:f=w330:T2)
            n164 = local write "State"(w330) -> ()
          }
        }
      }
    }
  }
  "error out" <- w4
